vi "AuxFindProb.vi"(6 "camera?":bool, 7 "nruns":i32, 8 "error in":errorcluster, 9 "threshholds":cluster{"t1 pmt":i32, "t1 camera":i32}, 10 "camera weight img":dbl[][](array[numeric]), 11 "READOUT":T1) -> (0 "error out":errorcluster, 3 "prob":dbl)   [LabVIEW 2019]
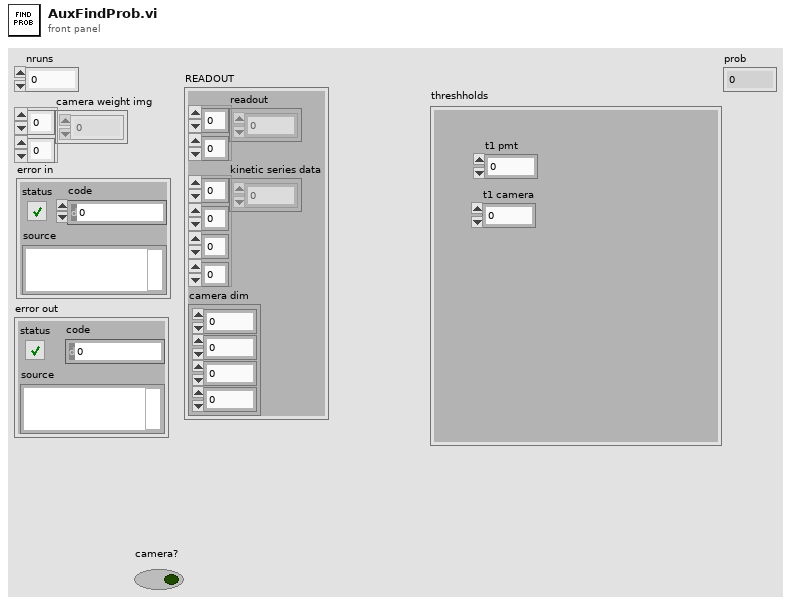
[diagram p1: front panel]
types:
  T1 = cluster{"readout":u32[][], "kinetic series data":i32[][][][], "camera dim":cluster{i32, i32, i32, i32}}
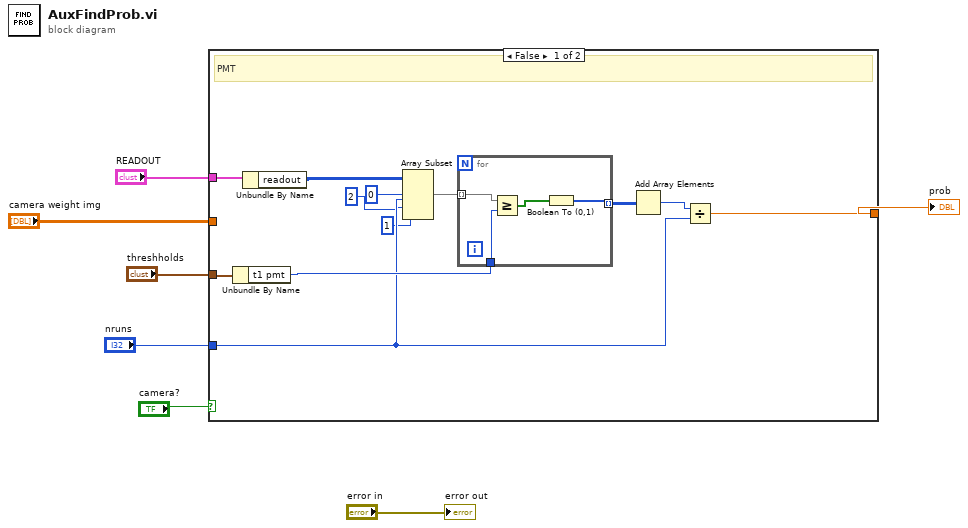
[diagram p0: block diagram]
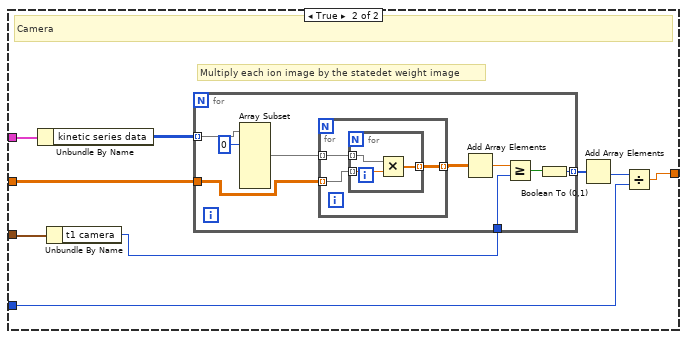
[diagram p2: hidden frame]
diagram:
  n1 = case shown="False" "camera?" {
    tunnel: "READOUT" -> [w19 w32]
    tunnel: "threshholds" -> [w18 w30]
    tunnel: "nruns" -> [w13 w24]
    tunnel: [w8 w25] -> w3
    tunnel: "camera weight img" -> [_ w29]
    frame False {
      # "PMT"
      n2 = Unbundle By Name(w18) -> ("t1 pmt"=w16:i32)
      n3 = Unbundle By Name(w19) -> ("readout"=w11:u32[][])
      n4 = Array Subset(array=w11, index (row)=0 ("index"), length (row)=w13, index (col)=2 ("index"), length (col)=1 ("length")) -> (w17:u32[][])
      n5 = for {
        tunnel: w17 -> [w23] mode=indexing
        tunnel: w16 -> [w22]
        tunnel: [w20] -> w15 mode=indexing
        n6 = Greater Or Equal?(x=w23, y=w22) -> (x >= y?=w21:bool[])
        n7 = Boolean To (0,1)(Boolean=w21) -> (0, 1=w20:i16[])
      }
      n8 = Add Array Elements(numeric array=w15) -> (sum=w14:i16)
      n9 = Divide(x=w14, y=w13) -> (x/y=w8:dbl)
    }
    frame True {
      # "Multiply each ion image by the statedet weight image"
      # "Camera"
      n10 = Unbundle By Name(w32) -> ("kinetic series data"=w31:i32[][][][])
      n11 = Unbundle By Name(w30) -> ("t1 camera"=w28:i32)
      n12 = for {
        tunnel: w31 -> [w41] mode=indexing
        tunnel: w29 -> [w38]
        tunnel: w28 -> [w35]
        tunnel: [w33] -> w27 mode=indexing
        n13 = Array Subset(array=w41, index (dim 0)=0 ("index")) -> (w39:i32[][][])  [unwired: 5 in]
        n14 = for {
          tunnel: w39 -> [w44] mode=indexing
          tunnel: w38 -> [w43] mode=indexing
          tunnel: [w42] -> w37 mode=indexing
          n15 = for {
            tunnel: w44 -> [w46] mode=indexing
            tunnel: w43 -> [w47] mode=indexing
            tunnel: [w45] -> w42 mode=indexing
            n16 = Multiply(x=w46, y=w47) -> (x*y=w45:dbl[])
          }
        }
        n17 = Add Array Elements(numeric array=w37) -> (sum=w36:dbl)
        n18 = Greater Or Equal?(x=w36, y=w35) -> (x >= y?=w34:bool)
        n19 = Boolean To (0,1)(Boolean=w34) -> (0, 1=w33:i16)
      }
      n20 = Add Array Elements(numeric array=w27) -> (sum=w26:i16)
      n21 = Divide(x=w26, y=w24) -> (x/y=w25:dbl)
    }
  }
  "prob" <- w3
  "error out" <- "error in"
